vi "Client Begin Client Streaming Call.vi"(5 "Response Message Name":string, 6 "contextId":T1, 7 "Request Message Name":string, 8 "error in":errorcluster, 9 "timeout (ms)":i32=-1, 10 "Method Name":string, 11 "ClientID in":T1) -> (0 "error out":errorcluster, 2 "Call ID out":T1, 3 "ClientID out":T1)   [LabVIEW 2019, in "grpc-lvsupport.lvlib"]
uses:
  grpc-lvsupport.lvlib
  Shared/grpcId.ctl
  <vilib>/Utility/error.llb/Error Cluster From Error Code.vi
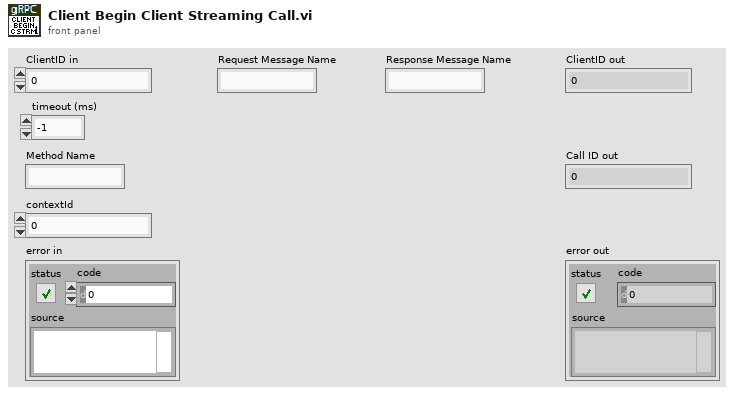
[diagram p1: front panel]
types:
  T1 = typedef "grpc-lvsupport.lvlib/grpcId.ctl" = u64
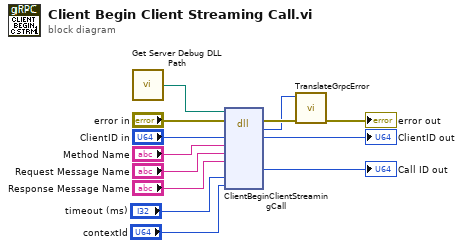
[diagram p0: block diagram]
diagram:
  n1 = call "Get Server Debug DLL Path.vi"() -> ("Server Debug DLL Path"=w11:path)
  n2 = dll-call lib="?" fn="ClientBeginClientStreamingCall"(path in=w11, error in="error in", "ClientId"="ClientID in", "methodName"="Method Name", "requestMessageName"="Request Message Name", "responseMessageName"="Response Message Name", "timeoutMs"="timeout (ms)", "contextId"="contextId") -> (error out=w12:errorcluster, "return type"=w3:i32, "ClientId"=→"ClientID out":u64, "callId"=→"Call ID out":u64)  [unwired: 7 in, 1 out]
  n3 = call "TranslateGrpcError.vi"("error in"=w12, "Error Code"=w3) -> ("error out"=→"error out":errorcluster)  [unwired: 9 in]
